vi "Query Channel Settings.vi"(8 "error in (no error)":errorcluster, 10 "ActiveChannel":i32, 11 "336XX in":refnum<class "336XX.lvclass">) -> (0 "error out":errorcluster, 3 "336XX out":refnum<class "336XX.lvclass">)   [LabVIEW 2019, in "336XX.lvlib" / "336XX.lvclass"]
uses:
  Library/336XX.lvclass
  C:/Users/Public/Documents/Development/builds/Instruments/FunctionGenerator.lvlibp/Library/FunctionGenerator.lvclass
  builds/Instruments/FunctionGenerator.lvlibp/Custom Controls/WaveformSettings.ctl
  builds/Instruments/FunctionGenerator.lvlibp/Custom Controls/WaveformMode.ctl
  builds/Instruments/FunctionGenerator.lvlibp/Accessors/Write Channel Settings.vi
  builds/Instruments/FunctionGenerator.lvlibp/Library/FunctionGenerator.lvclass
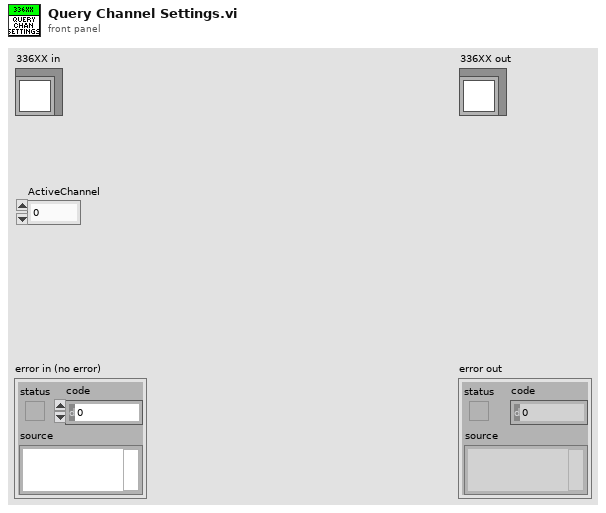
[diagram p1: front panel]
types:
  T1 = typedef "FunctionGenerator.lvlibp/FunctionGenerator.lvclass/WaveformSettings.ctl" = cluster{"Frequency":dbl, "Amplitude":dbl, "Offset":dbl, "Phase":dbl, "Symmetry":dbl, "Pulse Width":dbl, "Rise Time":dbl, "Fall Time":dbl, "Mode":T2, "Termination":enum16{"50_Ohm", "High_Z"}, "Output":bool}
  T2 = typedef "FunctionGenerator.lvlibp/FunctionGenerator.lvclass/WaveformMode.ctl" = enum16{"Sine", "Square", "Ramp", "Pulse", "Arbitrary", "Triangle", "Noise", "DC"}
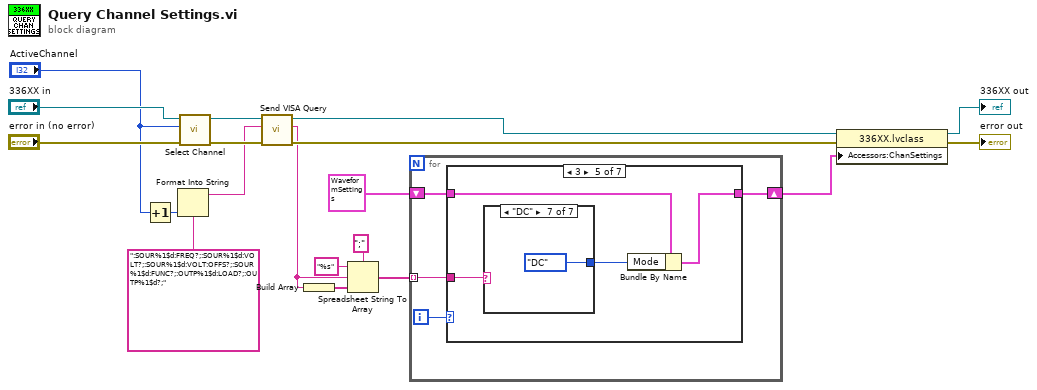
[diagram p0: block diagram]
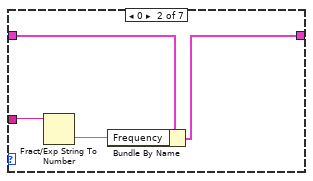
[diagram p3: hidden frame]
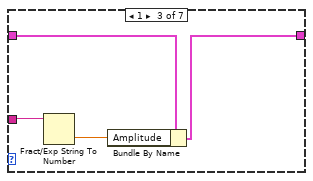
[diagram p4: hidden frame]
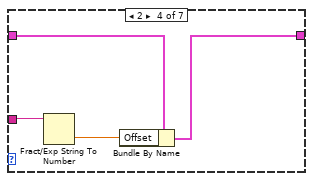
[diagram p5: hidden frame]
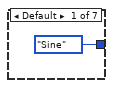
[diagram p6: hidden frame]
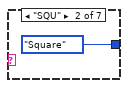
[diagram p7: hidden frame]
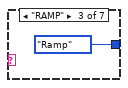
[diagram p8: hidden frame]
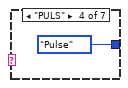
[diagram p9: hidden frame]
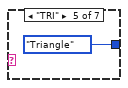
[diagram p10: hidden frame]
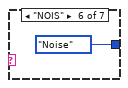
[diagram p11: hidden frame]
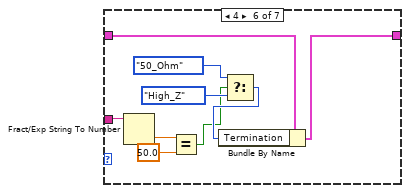
[diagram p12: hidden frame]
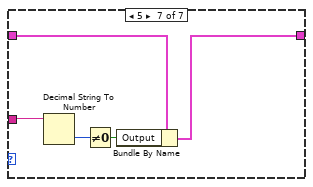
[diagram p13: hidden frame]
diagram:
  n1 = Increment(x="ActiveChannel") -> (x+1=w1:i32)
  n2 = Format Into String(format string=":SOUR%1$d:FREQ?;:SOUR%1$d:VOLT?;:SOUR%1$d:VOLT:OFFS?;:SOUR%1$d:FUNC?;:OUTP%1$d:LOAD?;:OUTP%1$d?;", w1) -> (resulting string=w12:string)  [unwired: 2 in, 1 out]
  n3 = call "Select Channel.vi"("error in (no error)"="error in (no error)", "Active Channel"="ActiveChannel", "FunctionGenerator in"="336XX in") -> ("error out"=w13:errorcluster, "FunctionGenerator out"=w14:refnum<class "336XX.lvclass">)  [unwired: 7 in]
  n4 = call "Send VISA Query.vi"("error in (no error)"=w13, "Command"=w12, "336XX in"=w14) -> ("error out"=w11:errorcluster, "Response"=w6:string, "336XX out"=w10:refnum<class "336XX.lvclass">)  [unwired: 6 in]
  n5 = Build Array(w6) -> (w9:string[])
  n6 = Spreadsheet String To Array(delimiter (Tab)=";", format string="%s", spreadsheet string=w6, array type (2D Dbl)=w9) -> (array=w5:string[])
  n7 = for {
    tunnel: w5 -> [w20] mode=indexing
    shift-right: [w21] -> w3
    shift-left: T1 {"Frequency"=0.0, "Amplitude"=0.0, "Offset"=0.0, "Phase"=0.0, "Symmetry"=0.0, "Pulse Width"=0.0, "Rise Time"=0.0, "Fall Time"=0.0, "Mode"=enum."Sine", "Termination"=enum."50_Ohm", "Output"=FALSE} ("FunctionGenerator:Settings:ChanSettings") -> [w22]
    i -> [w23]
    n8 = case shown="3" w23 {
      tunnel: w22 -> [w24 w28 w32 w36 w40 w56 w61]
      tunnel: [w24 w27 w31 w35 w39 w55 w60] -> w21
      tunnel: w20 -> [_ w26 w30 w34 w38 w54 w59]
      frame Default {
      }
      frame 0 {
        n9 = Fract/Exp String To Number(string=w26) -> (number=w25:dbl)  [unwired: 3 in, 1 out]
        n10 = Bundle By Name(cluster=w28, "Frequency"=w25) -> (w27:T1)
      }
      frame 1 {
        n11 = Fract/Exp String To Number(string=w30) -> (number=w29:dbl)  [unwired: 3 in, 1 out]
        n12 = Bundle By Name(cluster=w32, "Amplitude"=w29) -> (w31:T1)
      }
      frame 2 {
        n13 = Fract/Exp String To Number(string=w34) -> (number=w33:dbl)  [unwired: 3 in, 1 out]
        n14 = Bundle By Name(cluster=w36, "Offset"=w33) -> (w35:T1)
      }
      frame 3 {
        n15 = case shown="\"DC\"" w38 {
          tunnel: [WaveformMode."Sine" ("Mode") WaveformMode."Square" ("Mode") WaveformMode."Ramp" ("Mode") WaveformMode."Pulse" ("Mode") WaveformMode."Triangle" ("Mode") WaveformMode."Noise" ("Mode") WaveformMode."DC" ("Mode")] -> w37
          frame Default {
          }
          frame "SQU" {
          }
          frame "RAMP" {
          }
          frame "PULS" {
          }
          frame "TRI" {
          }
          frame "NOIS" {
          }
          frame "DC" {
          }
        }
        n16 = Bundle By Name(cluster=w40, "Mode"=w37) -> (w39:T1)
      }
      frame 4 {
        n17 = Fract/Exp String To Number(string=w54) -> (number=w51:dbl)  [unwired: 3 in, 1 out]
        n18 = Equal?(x=w51, y=50.0) -> (x = y?=w48:bool)
        n19 = Select(t=enum16{"50_Ohm", "High_Z"}."50_Ohm" ("Termination"), s=w48, f=enum16{"50_Ohm", "High_Z"}."High_Z" ("Termination")) -> (s? t:f=w49:enum16{"50_Ohm", "High_Z"})
        n20 = Bundle By Name(cluster=w56, "Termination"=w49) -> (w55:T1)
      }
      frame 5 {
        n21 = Decimal String To Number(string=w59) -> (number=w58:i32)  [unwired: 2 in, 1 out]
        n22 = Not Equal To 0?(x=w58) -> (x != 0?=w57:bool)
        n23 = Bundle By Name(cluster=w61, "Output"=w57) -> (w60:T1)
      }
    }
  }
  n24 = property class="336XX.lvclass"(reference=w10, error in=w11, "Accessors:ChanSettings"=w3) -> (reference out=→"336XX out":refnum<class "336XX.lvclass">, error out=→"error out":errorcluster)
